vi "LSMcontroller_v66_improvedwfhandling.vi"() -> ()   [LabVIEW 2015] (continued)
  out "Patch readout":dbl[][](graph)=[[-19.129690948880636, -18.936502231865173, -19.129690948880636, -19.065294709927485, -19.065294709927485, -19.097492829410562, -19.065294709927485, -19.000898470922337, -19.065294709927485, -19.065294709927485, -19.097492829410562, -19.129690948880636, -19.065294709927485, -19.22628530721287, -19.065294709927485, -19.033096590431416, -19.000898470922337, -19.129690948880636, -19.065294709927485, -19.000898470922337, -19.097492829410562, -19.097492829410562, -19.129690948880636, -19.097492829410562, -19.065294709927485, -19.19408718778179, -18.96870035140026, -19.033096590431416, -19.097492829410562, -19.033096590431416, -19.065294709927485, -19.065294709927485, -19.129690948880636, -19.097492829410562, -19.129690948880636, -19.16188906833771, -19.065294709927485, -19.065294709927485, -19.16188906833771, -19.16188906833771, -19.065294709927485, -19.129690948880636, -19.097492829410562, -19.033096590431416, -19.065294709927485, -19.129690948880636, -19.065294709927485, -19.033096590431416, -19.033096590431416, -19.129690948880636, -19.19408718778179, -19.065294709927485, -9.148273285922594, -9.212669532972436, -9.180471409454158, -9.083877038819596, -9.148273285922594, -9.148273285922594, -9.083877038819596, -9.148273285922594, -9.180471409454158, -9.180471409454158, -9.180471409454158, -9.212669532972436, -9.212669532972436, -9.180471409454158, -9.212669532972436, -9.11607516237774, -9.244867656477426, -9.11607516237774, -9.212669532972436, -9.244867656477426, -9.244867656477426, -9.11607516237774, -9.148273285922594, -9.212669532972436, -9.148273285922594, -9.212669532972436, -9.212669532972436, -9.180471409454158, -9.180471409454158, -9.277065779969131, -9.309263903447553, -9.244867656477426, -9.180471409454158, -9.180471409454158, -9.148273285922594, -9.244867656477426, -9.212669532972436, -9.244867656477426, -9.083877038819596, -9.212669532972436, -9.277065779969131, -9.244867656477426, -9.180471409454158, -9.11607516237774, -9.180471409454158, -9.212669532972436, -9.212669532972436, -9.212669532972436, -9.11607516237774, -9.180471409454158, -19.065294709927485, -19.097492829410562, -19.097492829410562, -19.16188906833771, -19.16188906833771, -19.033096590431416, -19.065294709927485, -19.129690948880636, -19.129690948880636, -19.097492829410562, -19.033096590431416, -19.258483426630953, -19.129690948880636, -19.033096590431416, -19.097492829410562, -19.129690948880636, -19.097492829410562, -19.19408718778179, -19.16188906833771, -19.097492829410562, -19.033096590431416, -19.000898470922337, -19.065294709927485, -19.16188906833771, -19.129690948880636, -19.129690948880636, -19.065294709927485, -19.033096590431416, -19.097492829410562, -19.097492829410562, -19.097492829410562, -18.96870035140026, -19.097492829410562, -19.19408718778179, -19.097492829410562, -19.065294709927485, -19.097492829410562, -19.129690948880636, -19.16188906833771, -19.033096590431416, -19.065294709927485, -19.129690948880636, -19.129690948880636, -19.065294709927485, -19.065294709927485, -19.033096590431416, -19.16188906833771, -19.097492829410562, -19.19408718778179, -19.000898470922337, -9.148273285922594, -9.148273285922594, -9.148273285922594, -9.019480791663437, -9.180471409454158, -9.277065779969131, -9.148273285922594, -9.148273285922594, -9.180471409454158, -9.180471409454158, -9.11607516237774, -9.180471409454158, -9.180471409454158, -9.11607516237774, -9.083877038819596, -9.341462026912685, -9.180471409454158, -9.11607516237774, -9.11607516237774, -9.212669532972436, -9.11607516237774, -9.11607516237774, -9.083877038819596, -9.11607516237774, -9.180471409454158, -9.11607516237774, -9.11607516237774, -9.244867656477426, -9.180471409454158, -9.180471409454158, -9.244867656477426, -9.180471409454158, -9.180471409454158, -9.180471409454158, -9.180471409454158, -9.180471409454158, -9.148273285922594, -9.11607516237774, -9.180471409454158, -9.212669532972436, -9.180471409454158, -9.148273285922594, -9.083877038819596, -9.11607516237774, -9.180471409454158, -9.148273285922594, -9.148273285922594, -9.148273285922594, -9.212669532972436, -9.11607516237774, -19.000898470922337, -19.065294709927485, -19.097492829410562, -19.129690948880636, -19.097492829410562, -18.936502231865173, -18.96870035140026, -19.097492829410562, -19.065294709927485, -19.097492829410562, -19.22628530721287, -19.065294709927485, -19.000898470922337, -19.000898470922337, -19.16188906833771, -19.065294709927485, -18.96870035140026, -19.097492829410562, -19.129690948880636, -19.065294709927485, -19.097492829410562, -19.129690948880636, -19.129690948880636, -19.16188906833771, -19.129690948880636, -19.129690948880636, -19.065294709927485, -19.000898470922337, -19.065294709927485, -19.065294709927485, -19.129690948880636, -19.033096590431416, -19.129690948880636, -19.065294709927485, -19.129690948880636, -19.097492829410562, -18.96870035140026, -19.097492829410562, -19.097492829410562, -19.065294709927485, -19.097492829410562, -19.129690948880636, -19.000898470922337, -19.033096590431416, -19.097492829410562, -19.097492829410562, -19.033096590431416, -18.96870035140026, -19.000898470922337, -19.129690948880636, -9.019480791663437, -9.083877038819596, -9.11607516237774, -9.083877038819596, -9.148273285922594, -9.309263903447553, -9.148273285922594, -9.11607516237774, -9.180471409454158, -9.180471409454158, -9.148273285922594, -9.148273285922594, -9.212669532972436, -9.019480791663437, -9.180471409454158, -9.148273285922594, -9.212669532972436, -9.051678915248162, -9.180471409454158, -9.212669532972436, -9.148273285922594, -9.212669532972436, -9.148273285922594, -9.11607516237774, -9.180471409454158, -9.212669532972436, -9.11607516237774, -9.083877038819596, -9.180471409454158, -9.11607516237774, -9.148273285922594, -9.083877038819596, -9.244867656477426, -9.212669532972436, -9.11607516237774, -9.11607516237774, -9.11607516237774, -9.148273285922594, -9.11607516237774, -9.11607516237774, -9.148273285922594, -9.180471409454158, -9.180471409454158, -9.051678915248162, -9.083877038819596, -9.083877038819596, -9.244867656477426, -9.083877038819596, -9.051678915248162, -9.148273285922594, -19.065294709927485, -19.065294709927485, -19.000898470922337, -19.000898470922337, -19.097492829410562, -19.065294709927485, -19.000898470922337, -19.097492829410562, -19.097492829410562, -19.033096590431416, -19.033096590431416, -19.033096590431416, -19.000898470922337, -19.065294709927485, -18.936502231865173, -19.065294709927485, -19.129690948880636, -19.065294709927485, -19.033096590431416, -19.000898470922337, -19.033096590431416, -19.065294709927485, -19.033096590431416, -19.065294709927485, -19.065294709927485, -19.129690948880636, -19.065294709927485, -19.033096590431416, -19.097492829410562, -19.033096590431416, -19.033096590431416, -19.097492829410562, -19.065294709927485, -19.129690948880636, -19.000898470922337, -19.033096590431416, -19.065294709927485, -19.097492829410562, -19.000898470922337, -19.033096590431416, -19.033096590431416, -19.000898470922337, -19.033096590431416, -19.033096590431416, -19.033096590431416, -19.033096590431416, -19.16188906833771, -19.000898470922337, -19.065294709927485, -19.065294709927485, -9.212669532972436, -9.083877038819596, -9.051678915248162, -9.148273285922594, -9.148273285922594, -9.212669532972436, -9.148273285922594, -9.148273285922594, -9.11607516237774, -9.11607516237774, -9.11607516237774, -9.11607516237774, -9.083877038819596, -9.180471409454158, -9.083877038819596, -9.11607516237774, -9.11607516237774, -9.244867656477426, -9.083877038819596, -9.019480791663437, -9.083877038819596, -9.212669532972436, -9.148273285922594, -9.083877038819596, -9.11607516237774, -9.11607516237774, -9.083877038819596, -9.083877038819596, -9.083877038819596, -8.987282668065419, -9.083877038819596, -9.148273285922594, -9.180471409454158, -9.083877038819596, -9.11607516237774, -9.212669532972436, -9.212669532972436, -9.083877038819596, -9.180471409454158, -9.148273285922594, -9.180471409454158, -9.180471409454158, -9.212669532972436, -9.180471409454158, -9.180471409454158, -9.11607516237774, -9.180471409454158, -9.244867656477426, -9.148273285922594, -9.148273285922594, -19.097492829410562, -19.16188906833771, -19.097492829410562, -19.033096590431416, -19.097492829410562, -19.033096590431416, -19.065294709927485, -19.097492829410562, -19.065294709927485, -19.000898470922337, -19.000898470922337, -19.000898470922337, -19.000898470922337, -19.065294709927485, -19.097492829410562, -19.065294709927485, -19.033096590431416, -19.129690948880636, -19.19408718778179, -19.097492829410562, -19.033096590431416, -19.16188906833771, -19.097492829410562, -19.16188906833771, -19.129690948880636, -19.065294709927485, -19.065294709927485, -19.000898470922337, -19.16188906833771, -19.129690948880636, -19.065294709927485, -19.097492829410562, -19.129690948880636, -19.19408718778179, -19.097492829410562, -19.129690948880636, -19.097492829410562, -19.097492829410562, -19.16188906833771, -19.033096590431416, -19.097492829410562, -19.129690948880636, -19.033096590431416, -19.097492829410562, -19.129690948880636, -19.22628530721287, -19.16188906833771, -19.065294709927485, -19.033096590431416, -19.097492829410562, -9.180471409454158, -9.180471409454158, -9.277065779969131, -9.244867656477426, -9.212669532972436, -9.11607516237774, -9.083877038819596, -9.11607516237774, -9.244867656477426, -9.019480791663437, -9.148273285922594, -9.083877038819596, -9.148273285922594, -9.051678915248162, -9.148273285922594, -9.019480791663437, -9.180471409454158, -9.148273285922594, -9.148273285922594, -9.212669532972436, -9.083877038819596, -8.987282668065419, -9.11607516237774, -9.212669532972436, -9.244867656477426, -9.083877038819596, -9.083877038819596, -9.083877038819596, -9.148273285922594, -9.148273285922594, -9.11607516237774, -9.212669532972436, -9.148273285922594, -9.148273285922594, -9.180471409454158, -9.019480791663437, -9.148273285922594, -9.180471409454158, -9.083877038819596, -9.083877038819596, -9.180471409454158, -9.212669532972436, -9.083877038819596, -9.11607516237774, -9.180471409454158, -9.180471409454158, -9.11607516237774, -9.180471409454158], [-35.779977141471754, -40.28771474745375, -34.49205210635021, -34.1700708472335, -34.81403336533239, -37.067902174441265, -37.71186469011919, -35.45799588289315, -36.423939658225486, -35.136014624180035, -37.067902174441265, -41.253658516736806, -35.779977141471754, -35.136014624180035, -40.609696004015795, -41.89762102892044, -34.49205210635021, -35.45799588289315, -35.779977141471754, -35.779977141471754, -36.74592091640061, -32.88214580942104, -38.677808462627745, -35.136014624180035, -35.45799588289315, -37.71186469011919, -34.49205210635021, -34.81403336533239, -36.101958399915866, -37.71186469011919, -39.64375223392652, -38.35582720525932, -37.067902174441265, -39.96573349075733, -35.136014624180035, -39.64375223392652, -40.28771474745375, -38.033845947756475, -32.23818328970733, -36.74592091640061, -35.45799588289315, -34.49205210635021, -34.49205210635021, -40.609696004015795, -37.38988343234745, -34.49205210635021, -34.49205210635021, -37.71186469011919, -39.64375223392652, -39.64375223392652, -33.84808958798223, -34.81403336533239, 678.0528204855508, 1131.0810610228193, 502.25090087551973, 199.266378015621, 75.94752772468436, 25.074483129972915, 3.1797561257887312, -5.5137382458773425, -15.817138854881982, -15.817138854881982, -17.105063921275384, -19.68091404758065, -19.68091404758065, -16.78308265487962, -19.68091404758065, -15.49515758794595, -13.88525125123923, -14.529213786327267, -18.071007719652435, -18.392988985508072, -17.105063921275384, -16.461101388348812, -13.56326998349251, -18.071007719652435, -17.74902645366178, -17.105063921275384, -20.9688391074937, -12.275344911154063, -18.071007719652435, -19.036951516814337, -18.071007719652435, -18.714970251228706, -15.49515758794595, -15.49515758794595, -19.036951516814337, -15.49515758794595, -21.612801636640594, -12.919307447593619, -11.953363642731512, -18.071007719652435, -15.173176320874825, -13.56326998349251, -15.817138854881982, -15.49515758794595, -17.74902645366178, -18.714970251228706, -13.88525125123923, -15.173176320874825, -18.714970251228706, -15.173176320874825, -733.5130643686014, -1187.5061495938146, -557.3894460524117, -254.08323998283743, -130.76444258972012, -71.84187725332792, -51.87903989910548, -42.863564796188484, -39.64375223392652, -38.677808462627745, -39.32177097696133, -41.89762102892044, -38.999789719861745, -33.20412706907601, -37.38988343234745, -37.38988343234745, -35.779977141471754, -38.35582720525932, -36.423939658225486, -33.84808958798223, -37.067902174441265, -33.52610832859641, -32.23818328970733, -37.38988343234745, -38.033845947756475, -34.81403336533239, -39.32177097696133, -40.28771474745375, -35.136014624180035, -37.067902174441265, -38.35582720525932, -34.1700708472335, -36.423939658225486, -35.779977141471754, -34.49205210635021, -37.71186469011919, -36.74592091640061, -33.84808958798223, -35.45799588289315, -34.81403336533239, -33.52610832859641, -36.101958399915866, -38.999789719861745, -44.15148981733241, -35.779977141471754, -34.81403336533239, -32.88214580942104, -41.89762102892044, -34.49205210635021, -33.20412706907601, 674.8330046967607, 1133.9788972951085, 500.9629748915052, 201.52024753339165, 76.59149033645211, 24.43052056204702, -0.6840191627033408, -12.597326179441428, -12.275344911154063, -10.987419836652661, -14.529213786327267, -22.578745429349105, -19.036951516814337, -12.919307447593619, -17.74902645366178, -15.173176320874825, -16.461101388348812, -20.324876577807075, -13.241288715610644, -14.8511950536686, -14.529213786327267, -13.88525125123923, -15.49515758794595, -19.036951516814337, -19.036951516814337, -12.597326179441428, -21.612801636640594, -24.83261427428173, -16.461101388348812, -12.597326179441428, -17.74902645366178, -15.49515758794595, -14.20723251885081, -17.105063921275384, -15.817138854881982, -16.139120121682932, -20.324876577807075, -17.74902645366178, -17.105063921275384, -16.139120121682932, -19.35893278226498, -17.105063921275384, -20.00289531276134, -18.392988985508072, -17.74902645366178, -13.56326998349251, -16.78308265487962, -21.29082037213461, -20.646857842717857, -12.597326179441428, -730.615235463241, -1184.6083220554708, -557.3894460524117, -256.01512699731944, -130.12048015097793, -78.92546457817109, -55.09885241038406, -42.21960228481076, -41.5756397728958, -38.033845947756475, -35.45799588289315, -36.74592091640061, -34.81403336533239, -39.32177097696133, -34.1700708472335, -35.45799588289315, -38.033845947756475, -34.81403336533239, -38.35582720525932, -37.067902174441265, -34.49205210635021, -35.45799588289315, -38.999789719861745, -39.32177097696133, -41.5756397728958, -37.067902174441265, -33.84808958798223, -37.71186469011919, -37.38988343234745, -35.136014624180035, -39.64375223392652, -34.81403336533239, -38.999789719861745, -36.101958399915866, -38.35582720525932, -38.35582720525932, -38.033845947756475, -41.5756397728958, -40.93167726044347, -33.84808958798223, -33.52610832859641, -31.916202029648574, -37.38988343234745, -37.38988343234745, -32.23818328970733, -38.35582720525932, -36.423939658225486, -38.677808462627745, -34.1700708472335, -34.49205210635021, 678.6967836451707, 1128.8271883760178, 499.35306741486363, 196.6905271466478, 77.55743425513697, 26.040426982883794, 1.5698497532110507, -12.275344911154063, -15.817138854881982, -11.631382374173768, -12.275344911154063, -18.071007719652435, -16.78308265487962, -20.00289531276134, -20.9688391074937, -16.461101388348812, -19.036951516814337, -16.461101388348812, -16.139120121682932, -19.35893278226498, -16.78308265487962, -19.68091404758065, -13.56326998349251, -15.173176320874825, -16.461101388348812, -21.612801636640594, -18.071007719652435, -13.88525125123923, -17.105063921275384, -17.4270451875361, -13.241288715610644, -13.88525125123923, -20.324876577807075, -19.036951516814337, -17.4270451875361, -16.461101388348812, -21.612801636640594, -16.461101388348812, -19.036951516814337, -18.392988985508072, -13.241288715610644, -16.78308265487962, -20.646857842717857, -16.139120121682932, -13.241288715610644, -10.987419836652661, -13.88525125123923, -23.222707957147, -16.139120121682932, -17.4270451875361, -732.2251404118074, -1186.540207081943, -556.4235028932625, -250.21946594002904, -128.51057405181638, -80.8573520192037, -56.38677741114458, -43.82950856224784, -38.677808462627745, -35.136014624180035, -34.1700708472335, -38.033845947756475, -33.84808958798223, -37.067902174441265, -35.45799588289315, -38.999789719861745, -37.067902174441265, -38.999789719861745, -38.677808462627745, -41.89762102892044, -37.067902174441265, -35.779977141471754, -35.45799588289315, -36.423939658225486, -34.49205210635021, -34.1700708472335, -43.82950856224784, -37.38988343234745, -32.88214580942104, -36.74592091640061, -37.71186469011919, -33.20412706907601, -36.423939658225486, -34.1700708472335, -36.423939658225486, -38.677808462627745, -35.779977141471754, -38.35582720525932, -37.38988343234745, -35.45799588289315, -35.136014624180035, -27.086483112608153, -38.033845947756475, -40.93167726044347, -34.49205210635021, -38.35582720525932, -39.32177097696133, -39.64375223392652, -39.32177097696133, -37.38988343234745, 679.340746805411, 1135.910788150883, 504.50477135332426, 202.80817297522802, 79.1673407890343, 21.854670295792648, -3.5818506162647887, -11.309401105480822, -6.157700787998381, -12.275344911154063, -20.646857842717857, -17.105063921275384, -13.241288715610644, -16.139120121682932, -17.105063921275384, -19.036951516814337, -18.714970251228706, -16.461101388348812, -21.93478290101167, -14.8511950536686, -13.56326998349251, -17.105063921275384, -12.275344911154063, -14.20723251885081, -19.036951516814337, -16.139120121682932, -17.105063921275384, -19.68091404758065, -12.275344911154063, -19.68091404758065, -22.256764165247834, -16.461101388348812, -15.173176320874825, -17.74902645366178, -18.392988985508072, -15.817138854881982, -16.461101388348812, -22.256764165247834, -16.139120121682932, -15.49515758794595, -11.953363642731512, -18.714970251228706, -21.612801636640594, -17.74902645366178, -11.631382374173768, -16.139120121682932, -15.817138854881982, -17.74902645366178, -15.49515758794595, -11.953363642731512, -735.1229693120254, -1187.1841687566255, -553.5256734093635, -255.04918349065514, -131.08642380889358, -77.63753961481774, -57.67470240976262, -42.21960228481076, -37.067902174441265, -36.101958399915866, -39.96573349075733, -38.999789719861745, -33.84808958798223, -36.74592091640061, -38.35582720525932, -38.35582720525932, -38.35582720525932, -38.999789719861745, -35.45799588289315, -36.101958399915866, -38.999789719861745, -40.609696004015795, -35.136014624180035, -38.033845947756475, -42.54158354056677, -31.272239509127207, -39.64375223392652, -35.45799588289315, -31.916202029648574, -34.1700708472335, -39.64375223392652, -38.033845947756475, -31.5942207694552, -37.38988343234745, -40.28771474745375, -35.779977141471754, -34.81403336533239, -35.136014624180035, -35.45799588289315, -35.136014624180035, -37.067902174441265, -38.35582720525932, -36.423939658225486, -35.45799588289315, -35.45799588289315, -37.71186469011919, -38.677808462627745, -38.677808462627745, -38.35582720525932, -31.916202029648574, 679.6627283857648, 1130.7590792156293, 502.8948638684274, 203.4521356969947, 73.69365858783573, 23.142595427830134, 0.9258872051291477, -4.22581316001062, -12.597326179441428, -15.173176320874825, -18.714970251228706, -20.646857842717857, -16.461101388348812, -17.74902645366178, -15.49515758794595, -15.49515758794595, -16.139120121682932, -16.461101388348812, -15.817138854881982, -16.139120121682932, -19.036951516814337, -11.631382374173768, -12.597326179441428, -15.173176320874825, -18.071007719652435, -19.35893278226498, -19.036951516814337, -15.49515758794595, -18.714970251228706, -15.817138854881982, -20.00289531276134, -17.74902645366178, -16.78308265487962, -16.139120121682932, -13.88525125123923, -16.139120121682932, -19.35893278226498, -21.612801636640594, -12.275344911154063, -20.324876577807075, -18.714970251228706, -17.74902645366178, -12.597326179441428, -15.49515758794595, -17.74902645366178, -21.29082037213461, -12.275344911154063, -13.88525125123923]]
  in  "Vholding (mV)":sgl caption="Vhold (mV)" step=0.1 format="%_6g"
  in  "sealtest":bool
  in  "Current Clamp":bool
  out "Rpipette (MOhm)":dbl
  out "Sampling rate \ncurrent wf":dbl
  out "remDO":bool
  out "addDO":bool
  in  "refwf":u32(ring)=3 caption="reference waveforms to:" items=["X", "Y", "2P pockels cell", "640 AO", "488 AO", "532 AO", "Voltage to Patch", "Voltage to Zpos", "2p Shutter", "488 shutter", "camera trigger", "640 shutter", "LT timestamp", "640 blanking", "488 blanking", "532 blanking", "2P ODfilt trigger ", "LCVR red", "LCVR blue"]
  out "remAO":bool
  out "addAO":bool
  in  "Add AO wave":bool
  out "Analog Used Lines":tag[](array[tag])
  in  "Rem AO wave":bool
  in  "Add DO wave":bool
  in  "Build digital waveform tabs":enum32{"Simple", "Matlab"}(tab)
  out "not loadedDO":bool caption="not loaded"
  in  "Digital time offset (s)":dbl
  in  "Digital padding value":dbl
  in  "Digital phase (s)":dbl
  in  "Digital DC (%)":dbl=50.0
  in  "Digital Freq (Hz)":dbl=50.0
  in  "load changed DO wave":bool
  out "changeDO":bool
  out "not loadedDOml":bool caption="not loaded"
  in  "Matlab padding value DO":dbl caption="Matlab padding value"
  in  "Load Matlab Waveform DO":bool
  in  "Matlab waveform path DO":path caption="Matlab waveform path"
  out "changeDOmatlab":bool
  out "Digital Used Lines":tag[](array[tag])
  in  "Rem DO wave":bool
  out "Total Camera Frames":i32=-1
  out "Digital Lines Plot":digitalwaveform[](graph)
  out "Analog Lines Plot":waveform(dbl)[](graph)
  in  "Build analog waveform tabs":enum32{"Square", "Triangle", "Matlab"}(tab)
  out "not loaded":bool
  in  "padding value":dbl
  in  "Start amplitude (V)":dbl=1.0
  in  "Period (ms)":dbl=1000.0
  in  "DC (%)":dbl=100.0
  in  "Step size (V)":dbl=1.0
  in  "Baseline (V)":dbl
  in  "Cycles":dbl=5.0
  in  "Repeats":dbl=1.0
  in  "phase shift (ms)":dbl=1.0
  in  "Pulses":dbl=1.0
  in  "load changed AOsq":bool
  out "changeAOsq":bool
  in  "Tri padding value":dbl
  in  "Tri Phase (s)":dbl
  in  "Tri Repeats":dbl
  in  "Frequency":dbl
  in  "Offset (V)":dbl
  in  "Amplitude (V)":dbl
  out "changeAOtri":bool
  in  "load changed AOtri":bool
  out "not loadedtri":bool caption="not loaded"
  in  "Matlab padding value":dbl
  in  "Load Matlab Waveform":bool
  in  "Matlab waveform path":path
  out "changeAOmatlab":bool
  out "not loadedml":bool caption="not loaded"
  out "Digital Used Names":string[](array[string])
  out "Analog Used Names":string[](array[string])
  in  "AO channels":u32(ring)=3 items=["X", "Y", "2P pockels cell", "640 AO", "488 AO", "532 AO", "Voltage to Patch", "Voltage to Zpos"]
  in  "DO channels":u16(ring) items=["2p Shutter", "488 shutter", "camera trigger", "640 shutter", "LT timestamp", "640 blanking", "488 blanking", "532 blanking", "2P ODfilt trigger ", "LCVR red", "LCVR blue"]
  in  "Loaded settings":u16(ring) items=["miao_patch", "miao_patch2"]
  in  "Setting location":path=path "C:/Users/Labmember/Desktop/Temp Data/2015-04-07 (Neurons DIV7 retigabine)/150957_Dish1_Cell07_1p5OD_p2"
  in  "Nickname":string="Pulse1"
  in  "Add settings":bool
  in  "Rem setting":bool
  in  "Update settings":bool
  in  "Bin size":T6(ring)
  out "Histogram 2":u32[](graph)
  out "Integral count":u32
  out "Lifetime (ns)":dbl
  in  "Input Method":u16(ring) items=["Unbinned", "Binned"]
  out "Ch1Rate":i32(slide) scale=0.01..100000000.0 scale format="%.0e"
  out "SyncRate":i32(slide) scale=0.01..100000000.0 scale format="%.0e"
  out "Histogram":u32[](graph)
  in  "Ch1 Level":i32=300 min=0 max=800 step=10
  in  "Ch1 ZeroX":i32=10 min=0 max=20 step=1
  in  "Ch0 ZeroX":i32=10 min=0 max=20 step=1
  in  "Ch0 Level":i32=70 min=0 max=800 step=10
  out "Save tab":enum32{"withsave", "withoutsave"}(tab)
  in  "save\ndata":bool=TRUE
  in  "filename prefix":string
  out "data dir":path=path "C:/Users/Labmember/Desktop/Data/temp" caption="save folder for data of current measurement"
  in  "AI channels":i32[](listbox)=[4]
  in  "avpp":i32=1 caption="# averages\n per point" min=1 step=1
  in  "# of frames":i32=1 caption="# of samples" min=1 step=1
  out "Current Average":sgl=1.0
  # "Sampling"
  # "Dataset"
  # "Hardware controls"
  # "Stage Joystick"
  # "Manual Coordinates"
  # "ROI Coordinates"
  # "Manual Coordinates"
  # "ROI Coordinates"
  # "Z-Scan"
  # "Patch controls"
  # "Patch mode"
  # "resting potential:\nHEKcells: -20 to -40 mV\n(down to -70 mV offset to get gigaseal)\nNeurons: -70 mV"
  # "Patch mode"
  # "determine R,C"
  # "Set gains (OC gain must equal  'Gain' on HEKA!!)"
  # "input Voltage for voltage clamp and monitored output Voltage are always amplified by a factor 10 compared to voltage over pipette --> factor implemented outomatically in VC input, and in in display here, raw output data are saved"
  # "OCG has three modes \nwith different noise, bandwidth and feedback resistor characteristics\nLow gain: 0.005-0.2 -->large currents, loose patch, large cells --> CC input gain=10 pA/mV\nMedium gain 0.5-20 --> normal whole cell recordings --> CC input gain = 0.1 pA/mV\nHigh gain 50-2K --> single channel --> current clamp not possible"
  # "DON'T FORGET TO CLOSE PICOHARP\nDON'T FORGET TO TURN ON 1040"
  # "should be O(1)"
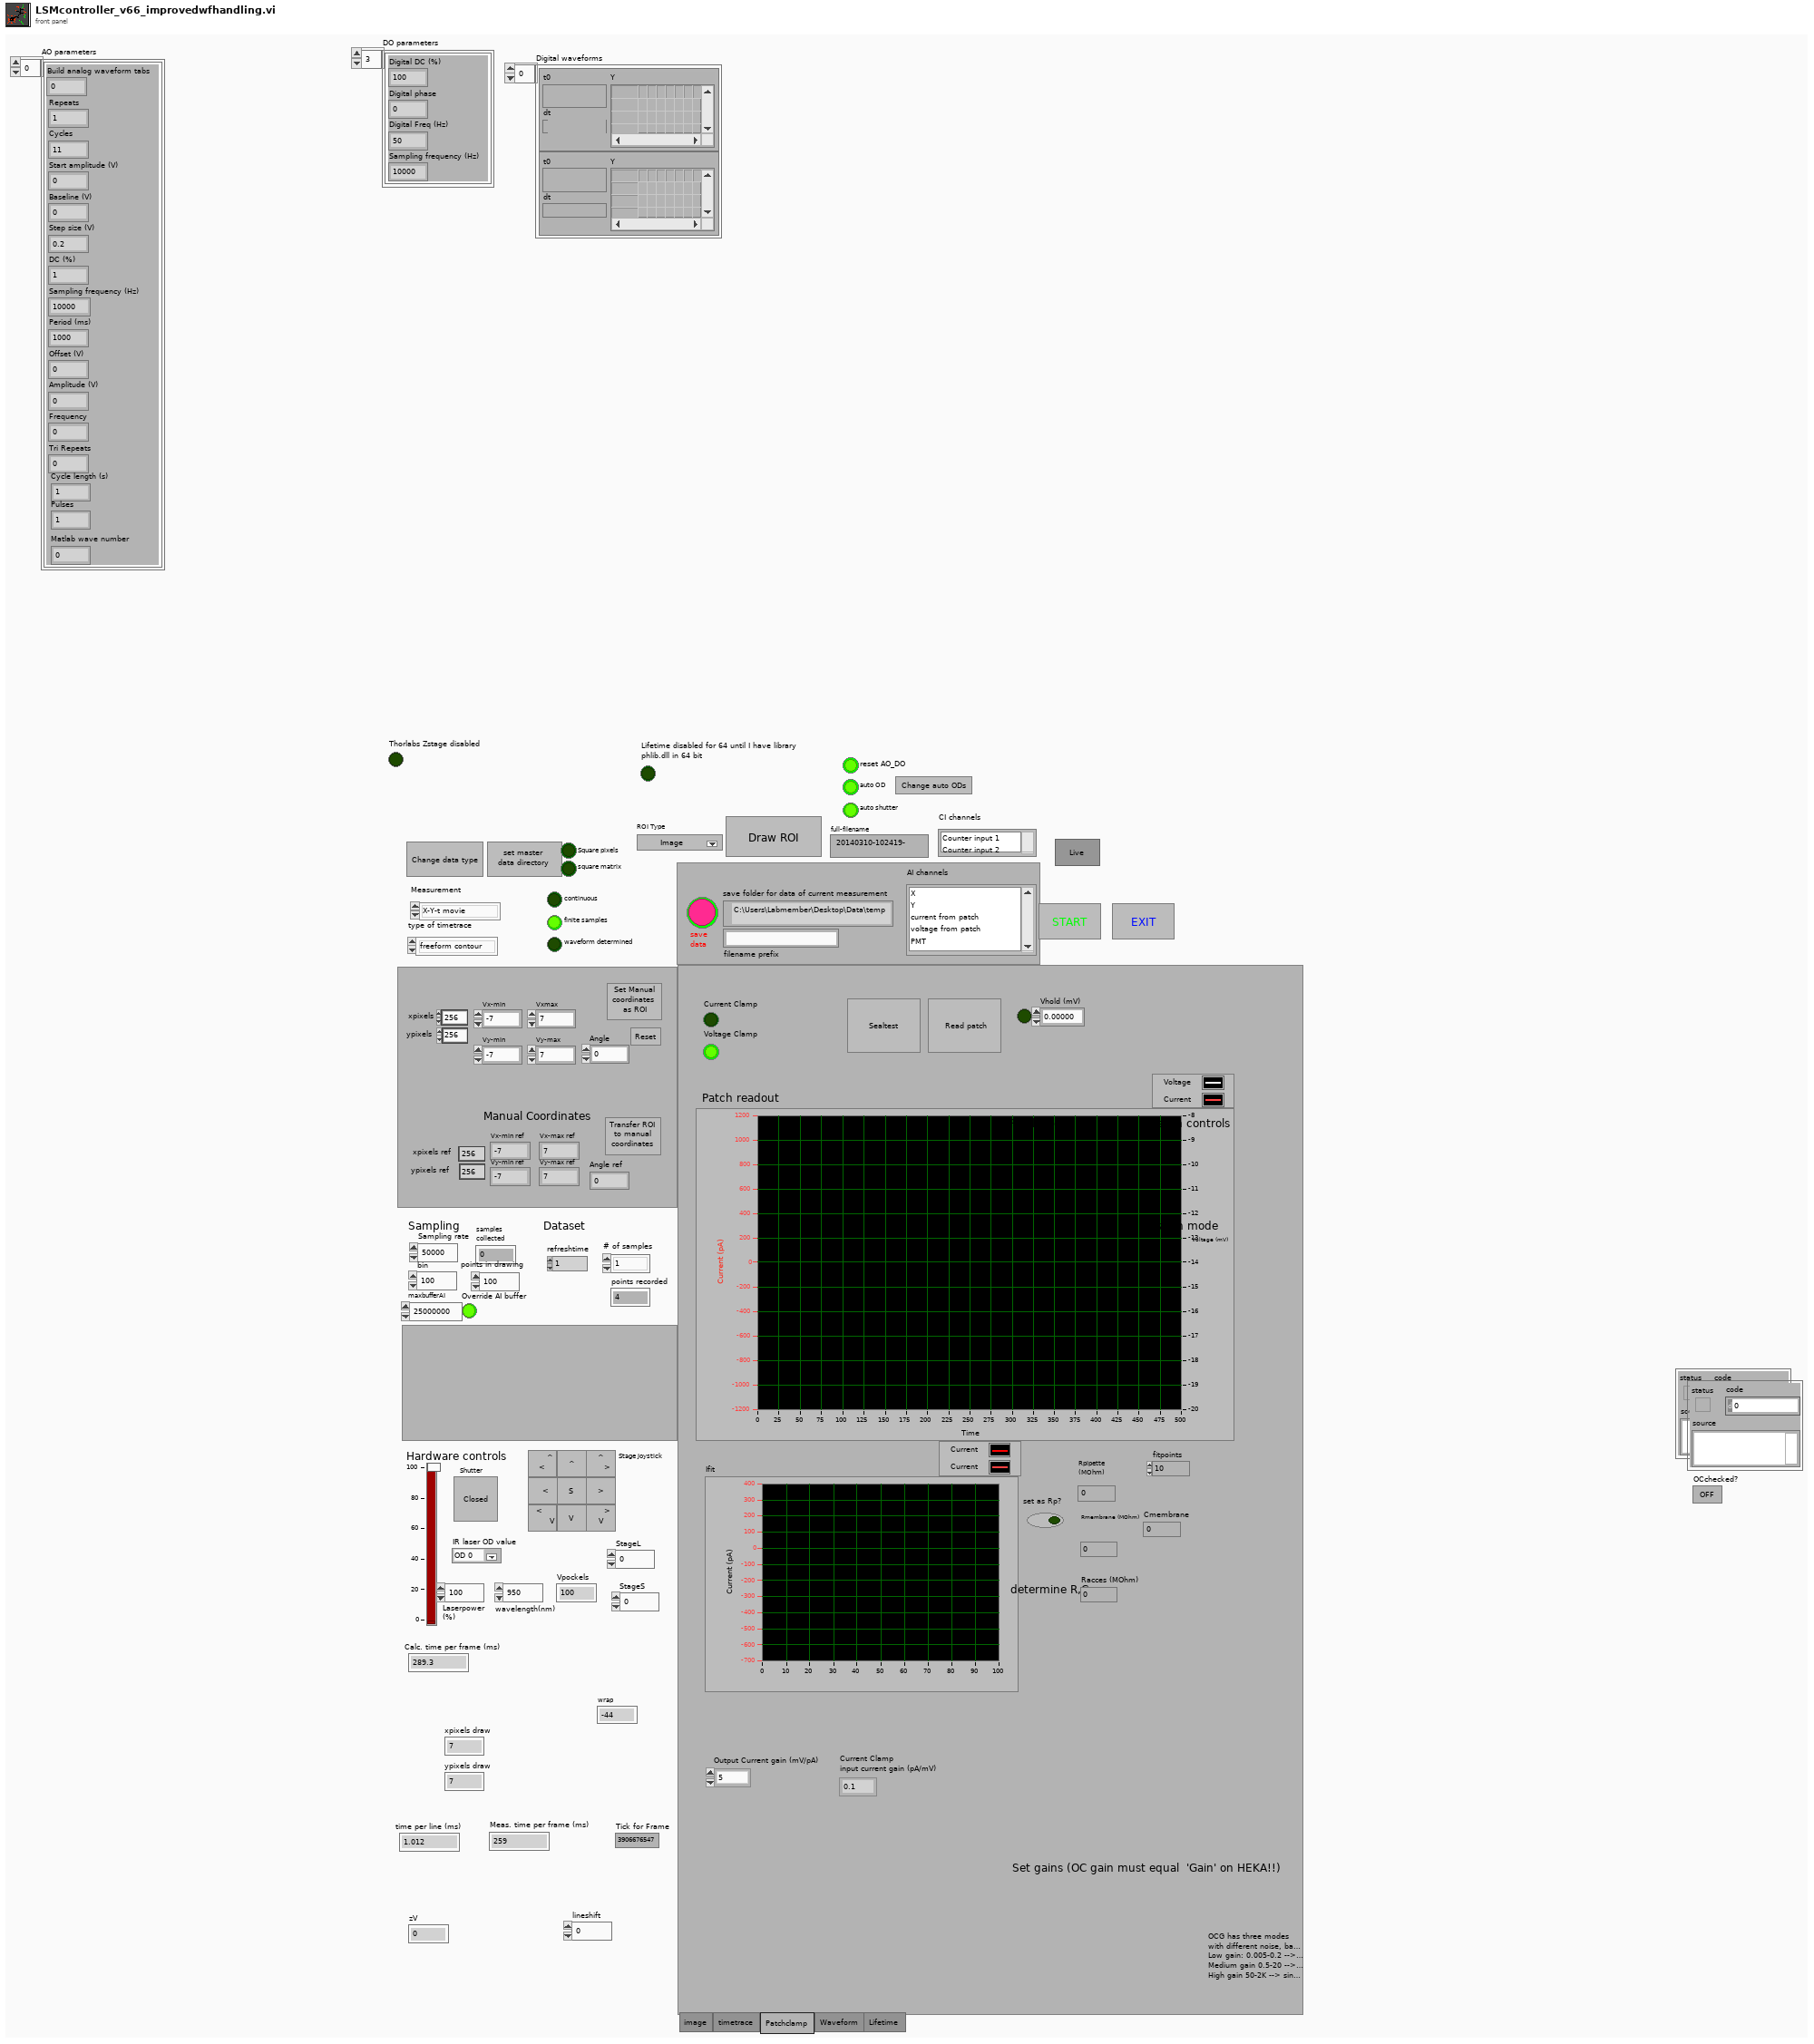
[diagram p1: front panel]
types:
  T1 = cluster{"Digital DC (%)":dbl, "Digital phase":dbl, "Digital Freq (Hz)":dbl, "Sampling frequency (Hz)":dbl}[]
  T2 = cluster{"Build analog waveform tabs":dbl, "Repeats":dbl, "Cycles":dbl, "Start amplitude (V)":dbl, "Baseline (V)":dbl, "Step size (V)":dbl, "DC (%)":dbl, "Sampling frequency (Hz)":dbl, "Period (ms)":dbl, "Offset (V)":dbl, "Amplitude (V)":dbl, "Frequency":dbl, "Tri Repeats":dbl, "Cycle length (s)":dbl, "Pulses":dbl, "Matlab wave number":dbl}[]
  T3 = enum16{"Point", "Resonant Ellipse", "Line", "freeform contour", "Fill Ellipse"}
  T4 = enum16{"X-Y-t movie", "X-Y-Z stack", "X-Y-Z-t movie", "linescan", "Timetrace", "Lifetime (point)", "Lifetime (scan)", "Lifetime (contour)"}
  T5 = enum32{"image", "timetrace", "Patchclamp", "Waveform", "Lifetime"}
  T6 = enum16{"1", "2", "4", "8", "16", "32", "64", "128"}
  T7 = enum8{"Enabled", "Disabled", "Disabled and Grayed Out"}
  T8 = enum16{"open", "replace", "create", "open or create", "replace or create", "replace or create with confirmation"}
  T9 = typedef "LVRectTypeDef.ctl" = cluster{"Left":i16, "Top":i16, "Right":i16, "Bottom":i16}
  T10 = cluster{"Xpixels":i32, "Vxminref":dbl, "Vxmaxref":dbl, "P":dbl, "Ypixels":i32, "Vyminref":dbl, "Vymaxref":dbl, "srate":sgl, "sAOxy":i32, "timeout":dbl, "type":string, "date":string, "time":string, "Colormap":u16, "Drawing Mode":u16, "Scanning Mode":u16, "square pixels":bool, "square matrix":bool, "Xpixels Img":i32, "Vx-min Img":dbl, "VX-max Img":dbl, "Ypixels Img":i32, "Vy-min Img":dbl, "Vy-max Img ":dbl, "Angle Img":dbl, "autoshutter":bool, "finite":bool, "cont":bool, "wavdet":bool, "measpoints":i32, "avpp":i32, "bufferAO":i32, "bufferAI":i32, "starttick":u32, "waveform":path, "Vx-ref":dbl, "Vy-ref":dbl, "refreshrate":dbl, "refreshbuffer":i32, "tt_cycles":i32, "motorref":refnum<k7>, "mirrorswitch":refnum<k7>, "sample mode":i32, "maxbufferAI":i32, "srateAODO":sgl, "bin":sgl, "Pel":sgl, "Angle draw":dbl, "srate Img":sgl, "ROIimg_plotbounds":T9, "auto OD":bool, "ODfilt":u16, "aAI":i32[], "aCI":i32[], "aAO":u32[], "aDO":u32[], "refwfsize":dbl, "Lifetime":bool, "Vz-Img":dbl, "Vz-ref":dbl, "Vz-reset":dbl, "AIoverride":bool}
  T11 = cluster{"StageS":i32, "StageL":i32, "currmeas data dir":path, "image OD":u16, "contour OD":u16, "point OD":u16, "AOlines":tag[], "AIlines":tag[], "CI lines":tag[], "DO lines":tag[], "AO names":string[], "CI names":string[], "AI names":string[], "DO names":string[], "CIextensions":string[], "AIextensions":string[], "Voltage to Ygalvo":i32, "Voltage to Xgalvo":i32, "Voltage to patch":i32, "640 shutter":i32, "2P shutter":i32, "LT timestamp":u32, "Vp":i32, "Ip":i32, "camera trigger":i32, "master data dir":path, "voltage to Zpos":i32, "Vto2P":i32, "640 AO":i32, "488 AO":i32, "532 AO":i32, "640TTL":u32, "488TTL":u32, "532TTL":u32, "Device 1 sampleclock out":tag, "Device 1 Starttrigger out":tag, "Device 2 sampleclock in":tag, "Device 2 StartTrigger in ":tag, "2PODTTL":u32, "488 shutter":u32, "LCVR red":u32, "LCVR blue":u32}
  T12 = enum16{"Left Button", "Center Button", "Right Button", "Window Close"}
  T13 = cluster{"VC":bool, "CC":bool, "CC_icg (pA/mv)":sgl, "VC_icg (mV/mV)":sgl, "OCG (mV/pA)":sgl, "OVG (mV/mV)":dbl, "Vhold (mV)":sgl, "holdon":bool}
  T14 = cluster{"AO parameters":cluster{"AOtab":dbl, "Repeats":dbl, "Cycles":dbl, "Start amplitude (V)":dbl, "Baseline (V)":dbl, "Step size (V)":dbl, "DC (%)":dbl, "Sampling frequency (Hz)":dbl, "Period (ms)":dbl, "Offset (V)":dbl, "Amplitude (V)":dbl, "Frequency":dbl, "Tri Repeats":dbl, "phase shift (ms)":dbl, "Pulses":dbl, "Matlab wave file":path, "Tri phase":dbl, "padding value":dbl}[], "DO parameters":cluster{"Digital DC (%)":dbl, "Digital phase":dbl, "Digital Freq (Hz)":dbl, "Sampling frequency (Hz)":dbl, "Digital time offset (s) ":dbl, "padding value":dbl, "matlab wave file":path, "DOtab":dbl}[]}
  T15 = cluster{"AOtab":dbl, "Repeats":dbl, "Cycles":dbl, "Start amplitude (V)":dbl, "Baseline (V)":dbl, "Step size (V)":dbl, "DC (%)":dbl, "Sampling frequency (Hz)":dbl, "Period (ms)":dbl, "Offset (V)":dbl, "Amplitude (V)":dbl, "Frequency":dbl, "Tri Repeats":dbl, "phase shift (ms)":dbl, "Pulses":dbl, "Matlab wave file":path, "Tri phase":dbl, "padding value":dbl}[]
  T16 = cluster{"AOtab":dbl, "Repeats":dbl, "Cycles":dbl, "Start amplitude (V)":dbl, "Baseline (V)":dbl, "Step size (V)":dbl, "DC (%)":dbl, "Sampling frequency (Hz)":dbl, "Period (ms)":dbl, "Offset (V)":dbl, "Amplitude (V)":dbl, "Frequency":dbl, "Tri Repeats":dbl, "phase shift (ms)":dbl, "Pulses":dbl, "Matlab wave file":path, "Tri phase":dbl, "padding value":dbl}
  T17 = cluster{"Digital DC (%)":dbl, "Digital phase":dbl, "Digital Freq (Hz)":dbl, "Sampling frequency (Hz)":dbl, "Digital time offset (s) ":dbl, "padding value":dbl, "matlab wave file":path, "DOtab":dbl}[]
  T18 = cluster{"Digital DC (%)":dbl, "Digital phase":dbl, "Digital Freq (Hz)":dbl, "Sampling frequency (Hz)":dbl, "Digital time offset (s) ":dbl, "padding value":dbl, "matlab wave file":path, "DOtab":dbl}
  T19 = cluster{"initialized":bool, "devidx":i32, "Ch0 Level":i32, "Ch0 ZeroX":i32, "Ch1 Level":i32, "Ch1 ZeroX":i32, "sync rate":i32, "resolution":i32, "acq time":i32, "acq rate":i32, "# bins":u32, "Bin size":enum16{"1", "2", "4", "8", "16", "32", "64", "128"}, "min photons":u32, "truncate":u32}
  T20 = cluster{"upleft":bool, "up":bool, "upright":bool, "right":bool, "downright":bool, "down":bool, "downleft":bool, "left":bool, "Bigsmall":bool, "E_stage":errorcluster}
  T21 = typedef "DialogType.ctl" = u16
  T22 = cluster{"AO parameters":cluster{"AOtab":dbl, "Repeats":dbl, "Cycles":dbl, "Start amplitude (V)":dbl, "Baseline (V)":dbl, "Step size (V)":dbl, "DC (%)":dbl, "Sampling frequency (Hz)":dbl, "Period (ms)":dbl, "Offset (V)":dbl, "Amplitude (V)":dbl, "Frequency":dbl, "Tri Repeats":dbl, "Cycle length (s)":dbl, "Pulses":dbl, "Matlab wave file":path, "Tri phase":dbl, "padding value":dbl}[]}
  T23 = cluster{"AOtab":dbl, "Repeats":dbl, "Cycles":dbl, "Start amplitude (V)":dbl, "Baseline (V)":dbl, "Step size (V)":dbl, "DC (%)":dbl, "Sampling frequency (Hz)":dbl, "Period (ms)":dbl, "Offset (V)":dbl, "Amplitude (V)":dbl, "Frequency":dbl, "Tri Repeats":dbl, "Cycle length (s)":dbl, "Pulses":dbl, "Matlab wave file":path, "Tri phase":dbl, "padding value":dbl}[]
  T24 = cluster{"AOtab":dbl, "Repeats":dbl, "Cycles":dbl, "Start amplitude (V)":dbl, "Baseline (V)":dbl, "Step size (V)":dbl, "DC (%)":dbl, "Sampling frequency (Hz)":dbl, "Period (ms)":dbl, "Offset (V)":dbl, "Amplitude (V)":dbl, "Frequency":dbl, "Tri Repeats":dbl, "Cycle length (s)":dbl, "Pulses":dbl, "Matlab wave file":path, "Tri phase":dbl, "padding value":dbl}
  T25 = cluster{"AO":refnum<k21>[], "E_AO":errorcluster[]}
  T26 = cluster{" AI":refnum<k21>, "E_AI":errorcluster, "header":dbl[]}
  T27 = cluster{"settings names":string[], "settings locations":path[]}
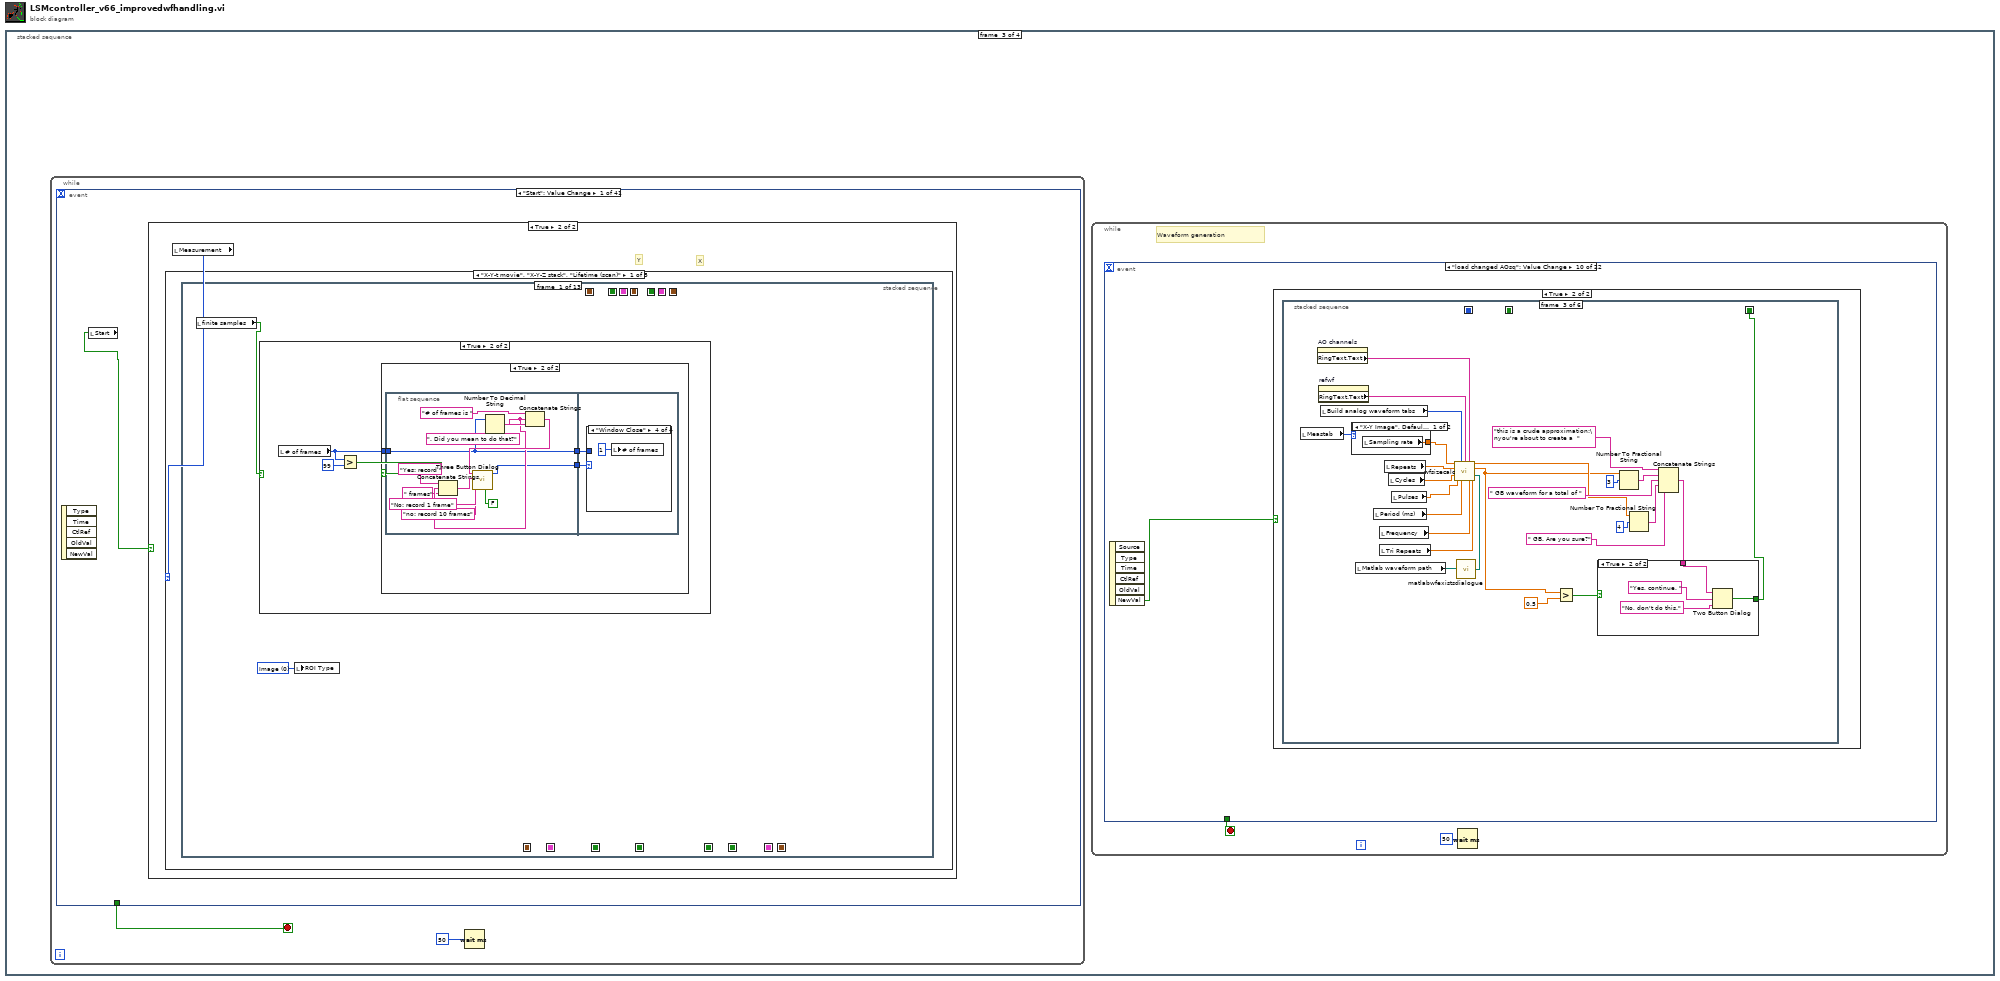
[diagram p0: block diagram]
diagram:
  n1 = stacked-sequence {
    frame #0 {
      "OCchecked?" <- FALSE ("Boolean")
    }
    frame #1 {
      w15 = u16 0 items=["Rectangle", "Circle", "Freeform Boundary", "Freeform Interior"] ("ROI Type")
      w24 = FALSE ("Value (Signaling)")
      # "Look in disabled \nchannelselect example next to this\nto understand how channels get propagated \nthrough the progam\n\nthe configuration file contains all\navailable channels in an array.\nat the start of the program lists of available \ninput channels and  menu rings of available output channels are loaded from here.\n\nif you add channels to record from/output to, make sure to expand the channel array in config.\n\nOnce the lists and rings are loaded, items in the list can be selected via click and  shift-click.\nThe ao channels in the ring are added one by one, with a defined waveform.\n\nPropagating through the program in the 2p param buffers are only 4 arrays of numbers, which are the indices of the selected channels from the list in order. \nThus, the index in the active channels array DOES NOT tell you which channel it represents: the actual CONTENT/NUMBER at a particular index in the active channels arrays tells you which channel it represents, since that number is the index in the fixed channel array in config."
      n2 = stacked-sequence {
        frame #0 {
          n3 = call "lifetimeparameters.vi"("command"="clear") -> ()  [unwired: 1 in, 1 out]
          n4 = call "2pparameters.vi"("command"="clear") -> ()  [unwired: 1 in, 1 out]
        }
        frame #1 {
          w39 = TRUE ("auto shutter")
          n5 = call "2pparameters.vi"("command"="get") -> ("params out"=w41:T10)  [unwired: 1 in]
          n6 = Bundle By Name(cluster=w41, "autoshutter"=w39, "auto OD"=w39) -> (w40:T10)
          n7 = local write "auto shutter"(w39) -> ()
          n8 = local write "auto OD"(w39) -> ()
          n9 = call "2pparameters.vi"("Params in"=w40, "command"="set") -> ()  [unwired: 1 out]
        }
        frame #2 {
        }
        frame #3 {
          n10 = call "2pparameters.vi"("command"="get") -> ("params out"=w46:T10)  [unwired: 1 in]
          n11 = Bundle By Name(cluster=w46, "type"="X-Y-t movie") -> (w48:T10)
          n12 = call "2pparameters.vi"("Params in"=w48, "command"="set") -> ()  [unwired: 1 out]
        }
      }
      n13 = property on="Exit" class="Bool (strict)"("Val(Sgnl)"=w24) -> ()  [unwired: 2 in, 2 out]
      n14 = property on="Start" class="Bool (strict)"("Val(Sgnl)"=w24) -> ()  [unwired: 2 in, 2 out]
      n15 = property on="Stop" class="Bool (strict)"("Val(Sgnl)"=w24) -> ()  [unwired: 2 in, 2 out]
      n16 = property on="Start" class="Bool (strict)"("Visible"=TRUE, "DisabledEnum"=T7."Enabled" ("Disabled")) -> ()  [unwired: 2 in, 2 out]
      n17 = property on="ROI" class="Bool (strict)"("DisabledEnum"=T7."Enabled" ("Disabled")) -> ()  [unwired: 2 in, 2 out]
      n18 = property on="ROI" class="Bool (strict)"("Value"=FALSE ("ROI")) -> ()  [unwired: 2 in, 2 out]
      n19 = property on="ROI" class="Bool (strict)"("Visible"=TRUE) -> ()  [unwired: 2 in, 2 out]
      n20 = local read "Measurement"() -> (w12:T4)
      n21 = flat-sequence {
        frame #0 {
          n22 = call "configuration.vi"("command"="set") -> ()  [unwired: 2 in, 2 out]
        }
        frame #1 {
          w50 = u16 1 items=["OD 0"=1, "OD 0.5"=2, "OD 1"=3, "OD 2"=4, "OD 3"=5, "OD 4"=6] ("New ODfilt")
          n23 = call "configuration.vi"("command"="get") -> ("config out"=w53:T11)  [unwired: 2 in, 1 out]
          n24 = local read "ODfilt"() -> (w51:u16)
          n25 = Unbundle By Name(w53) -> ("master data dir"=→"data dir":path)
          n26 = call "filterwheelcontrol_nothorlabslib.vi"("Current OD filt"=w50, "New ODfilt"=w51) -> ()  [unwired: 1 in]
        }
        frame #2 {
          n27 = call "configuration.vi"("command"="get") -> ("config out"=w57:T11)  [unwired: 2 in, 1 out]
          n28 = Unbundle By Name(w57) -> ("AI names"=w56:string[], "CI names"=w55:string[])
          n29 = property on="AI channels" class="LstBox (strict)"("Item Names"=w56) -> ()  [unwired: 2 in, 2 out]
          n30 = property on="CI channels" class="LstBox (strict)"("Item Names"=w55) -> ()  [unwired: 2 in, 2 out]
        }
        frame #3 {
          n31 = call "configuration.vi"("command"="get") -> ("config out"=w66:T11)  [unwired: 2 in, 1 out]
          n32 = Unbundle By Name(w66) -> ("AO names"=w62:string[], "DO names"=w61:string[])
          n33 = call "fill channelselector from array.vi"("channel  names"=w62) -> ("channel selector string and values"=w64:cluster{"String":string, "Value":u16}[])
          n34 = Build Array (concatenate)(w62, w61) -> (w60:string[])
          n35 = call "fill channelselector from array.vi"("channel  names"=w61) -> ("channel selector string and values"=w63:cluster{"String":string, "Value":u16}[])
          n36 = property on="AO channels" class="Ring (strict)"("StringsAndValues[]"=w64) -> ()  [unwired: 2 in, 2 out]
          n37 = call "fill channelselector from array.vi"("channel  names"=w60) -> ("channel selector string and values"=w59:cluster{"String":string, "Value":u16}[])
          n38 = property on="DO channels" class="Ring (strict)"("StringsAndValues[]"=w63) -> ()  [unwired: 2 in, 2 out]
          n39 = property on="refwf" class="Ring (strict)"("StringsAndValues[]"=w59) -> ()  [unwired: 2 in, 2 out]
        }
        frame #4 {
          n40 = call "moveZ_V2.vi"("Z"=0.0) -> ()
        }
      }
      n41 = case shown="\"Lifetime (point)\", \"Lifetime (scan)\"" w12 {
        frame "Lifetime (point)", "Lifetime (scan)" {
          n42 = property on="Init" class="Bool (strict)"("Visible"=TRUE, "DisabledEnum"=T7."Enabled" ("Disabled")) -> ()  [unwired: 2 in, 2 out]
          n43 = property on="Start" class="Bool (strict)"("Visible"=FALSE, "DisabledEnum"=T7."Disabled and Grayed Out" ("Disabled")) -> ()  [unwired: 2 in, 2 out]
        }
        frame "X-Y-t movie", Default {
        }
      }
      n44 = call "seterrors.vi"("error IO"=errorcluster {"status"=FALSE, "code"=0, "source"=""}) -> ()
      n45 = property on="Stop" class="Bool (strict)"("Visible"=FALSE, "DisabledEnum"=T7."Disabled and Grayed Out" ("Disabled")) -> ()  [unwired: 2 in, 2 out]
      n46 = property on="Init" class="Bool (strict)"("Visible"=FALSE, "DisabledEnum"=T7."Disabled and Grayed Out" ("Disabled")) -> ()  [unwired: 2 in, 2 out]
      n47 = Current VI's Path() -> (path=w10:path)
      n48 = Strip Path(path=w10) -> (stripped path=w11:path)  [unwired: 1 out]
      n49 = Build Path(base path=w11, name or relative path="LaserControl.vi") -> (appended path=w9:path)
      n50 = call "loadcolormaps.vi"() -> ()  [unwired: 12 in]
      n51 = stacked-sequence {
        frame #0 {
          n52 = call "waveformsDObuffer.vi"("command"="clear") -> ()  [unwired: 1 in, 1 out]
          n53 = call "waveformsAObuffer.vi"("command"="clear") -> ()  [unwired: 1 in, 1 out]
        }
        frame #1 {
          n54 = call "Used AO lines.vi"() -> ("used AO names"=w27:string[], "used AO lines"=w29:tag[])  [unwired: 2 in]
          n55 = control-ref of="Analog Lines Plot"() -> (w28:refnum<vi>)
          n56 = local write "Analog Used Lines"(w29) -> ()
          n57 = local write "Analog Used Names"(w27) -> ()
          n58 = call "prepAOWaveplot.vi"("WaveformGraph in"=w28, "Analog Used Names"=w27) -> ()  [unwired: 1 in]
          n59 = control-ref of="Digital Lines Plot"() -> (w30:refnum<vi>)
          n60 = call "Used DO lines.vi"() -> ("used DO names"=w31:string[], "used DO lines"=w32:tag[])  [unwired: 2 in]
          n61 = local write "Digital Used Lines"(w32) -> ()
          n62 = local write "Digital Used Names"(w31) -> ()
          n63 = call "prepDOWaveplot.vi"("DigitalGraph in"=w30, "used DO names"=w31) -> ()  [unwired: 1 in]
        }
      }
      n64 = Open VI Reference(type specifier VI Refnum (for type only)=refnum<vi> refnum, vi path=w9, options=128) -> (vi reference=w2:refnum<vi>, error out=w6:errorcluster)  [unwired: 3 in]
      n65 = call-by-ref "Start Asynchronous Call"(reference=w2, error in=w6) -> (reference out=w7:refnum<vi>, error out=w5:errorcluster)  [unwired: 12 in]
      n66 = Close Reference(reference=w7, error in (no error)=w5) -> ()  [unwired: 1 out]
      n67 = disable-structure shown="Enabled" {
        frame Disabled {
          n68 = call "channelselectexample.vi"() -> ()  [unwired: 12 in]
        }
        frame Enabled {
        }
      }
      "ROI Type" <- w15
    }
    frame #2 {
      n69 = while {
        stop <- w2241 stop-if-true
        n70 = event shown="[0] \"Start\": Value Change" {
          selector: _ -> [_ _ _ _ _ _ _ _ _ _ _ _ _ _ _ _ _ _ _ _ _ _ _ _ _ _ _ _ _ _ _ _ _ _ _ _ _ _ _ _ _]
          dyn-events: _ -> [_ _ _ _ _ _ _ _ _ _ _ _ _ _ _ _ _ _ _ _ _ _ _ _ _ _ _ _ _ _ _ _ _ _ _ _ _ _ _ _ _]
          timeout: _ -> [_ _ _ _ _ _ _ _ _ _ _ _ _ _ _ _ _ _ _ _ _ _ _ _ _ _ _ _ _ _ _ _ _ _ _ _ _ _ _ _ _]
          tunnel: [_ _ _ _ _ _ _ _ _ _ _ _ _ _ _ _ _ _ _ _ _ _ _ _ _ _ _ _ _ _ _ _ _ _ _ _ _ _ _ _ "Exit"] -> w2241
          event "Start": Value Change {
            n71 = event-data() -> ()  [unwired: 1 in, 5 out]
            n72 = local read "Start"() -> (w2242:bool)
            n73 = case shown="True" w2242 {
              frame False {
              }
              frame True {
                # "X"
                # "Y"
                n74 = local read "Measurement"() -> (w2243:T4)
                n75 = case shown="\"X-Y-t movie\", \"X-Y-Z stack\", \"Lifetime (scan)\"" w2243 {
                  frame "X-Y-t movie", "X-Y-Z stack", "Lifetime (scan)" {
                    n76 = stacked-sequence {
                      seq-local: [_ w2285 _ _ _ _ _ _ _ _ _ _ _] -> [_ _ _ w3138 _ _ _ w3174 w3355 _ _ w3765 _]
                      seq-local: [_ w2283 _ _ _ _ _ _ _ _ _ _ _] -> [_ _ _ _ _ _ _ _ _ _ w3455 _ _]
                      seq-local: [_ w2282 _ _ _ _ _ _ _ _ _ _ _] -> [_ _ _ _ _ _ _ _ _ _ w3454 _ _]
                      seq-local: [_ w2281 _ _ _ _ _ _ _ _ _ _ _] -> [_ _ _ _ _ _ _ _ _ _ w3453 _ _]
                      seq-local: [_ w2280 _ _ _ _ _ _ _ _ _ _ _] -> [_ _ _ _ _ _ _ _ _ _ w3452 _ _]
                      seq-local: [_ w2279 _ _ _ _ _ _ _ _ _ _ _] -> [_ _ _ _ _ _ _ _ _ _ w3451 _ _]
                      seq-local: [_ w2278 _ _ _ _ _ _ _ _ _ _ _] -> [_ _ _ _ _ _ _ _ _ _ w3450 _ _]
                      seq-local: [_ w2277 _ _ _ _ _ _ _ _ _ _ _] -> [_ _ _ _ _ _ _ _ _ _ w3445 _ _]
                      seq-local: [_ w2276 _ _ _ _ _ _ _ _ _ _ _] -> [_ _ _ _ _ _ _ _ _ _ w3444 _ _]
                      seq-local: [_ w2275 _ _ _ _ _ _ _ _ _ _ _] -> [_ _ _ _ _ _ _ _ _ _ w3449 _ _]
                      seq-local: [_ w2274 _ _ _ _ _ _ _ _ _ _ _] -> [_ _ _ _ _ _ _ _ _ _ w3448 _ _]
                      seq-local: [_ w2272 _ _ _ _ _ _ _ _ _ _ _] -> [_ _ _ _ _ _ _ _ _ _ w3443 _ _]
                      seq-local: [_ w2273 _ _ _ _ _ _ _ _ _ _ _] -> [_ _ _ _ _ _ _ _ _ _ w3442 _ _]
                      seq-local: [_ w2271 _ _ _ _ _ _ _ _ _ _ _] -> [_ _ _ _ _ _ _ _ _ _ w3446 _ _]
                      seq-local: [_ w2270 _ _ _ _ _ _ _ _ _ _ _] -> [_ _ _ _ _ _ _ _ _ _ w3447 _ _]
                      frame #0 {
                        w2244 = u16 0 items=["Image", "Rectangle", "Circle", "Freeform Boundary", "Freeform Interior", "Ellipse Boundary", "Line"] ("ROI Type")
                        n77 = local read "finite samples"() -> (w2245:bool)
                        n78 = case shown="True" w2245 {
                          frame False {
                          }
                          frame True {
                            n79 = local read "# of frames"() -> (w2246:i32)
                            n80 = Greater?(x=w2246, y=99) -> (0:w2247:bool)
                            n81 = case shown="True" w2247 {
                              tunnel: w2246 -> [_ w2251]
                              frame False {
                              }
                              frame True {
                                n82 = flat-sequence {
                                tunnel: w2251 -> [w2252]
                                tunnel: [w2253] -> w2250
                                tunnel: [w2252] -> w2249
                                tunnel: w2250 -> [w2265]
                                tunnel: w2249 -> [w2264]
                                frame #0 {
                                n83 = Number To Decimal String(number=w2252) -> (decimal integer string=w2257:string)  [unwired: 1 in]
                                n84 = Concatenate Strings("Yes: record " ("Left Button Text (\"Yes\")"), w2257, " frames" ("string")) -> (w2258:string)
                                n85 = Concatenate Strings("# of frames is " ("message"), w2257, ". Did you mean to do that?" ("string")) -> (w2260:string)
                                n86 = call <vilib>:"Three Button Dialog.vi"("Allow user to close window? (TRUE)"=FALSE, "Right Button Text (\"Cancel\")"="no: record 10 frames" ("Right Button Text (\"Cancel\")"), "Center Button Text (\"No\")"="No: record 1 frame" ("Center Button Text (\"No\")"), "Left Button Text (\"Yes\")"=w2258, "message"=w2260) -> ("Which Button?"=w2253:T12)  [unwired: 6 in]
                                }
                                frame #1 {
                                n87 = case shown="\"Window Close\"" w2265 {
                                tunnel: w2264 -> [w2266 _ _ _]
                                frame "Left Button" {
                                n88 = local write "# of frames"(w2266) -> ()
                                }
                                frame "Center Button", Default {
                                n89 = local write "# of frames"(1 ("# of frames")) -> ()
                                }
                                frame "Right Button" {
                                n90 = local write "# of frames"(10 ("# of frames")) -> ()
                                }
                                frame "Window Close" {
                                n91 = local write "# of frames"(1 ("# of frames")) -> ()
                                }
                                }
                                }
                                }
                              }
                            }
                          }
                        }
                        n92 = local write "ROI Type"(w2244) -> ()
                      }
                      frame #1 {
                        # "change active waveform numbers array"
                        n93 = local read "save\ndata"() -> (w2284:bool)
                        n94 = Get Date/Time In Seconds() -> (seconds since 1Jan1904=w2286:timestamp)
                        n95 = case shown="True" w2284 {
                          tunnel: w2286 -> [w2287 w2289]
                          tunnel: [w2287 w2288] -> w2285
